vi "Create HTML.vi"(7 "FP Reference":refnum<class "Web Front Panel.lvclass">, 8 "error in (no error)":errorcluster, 10 "VI Identifier":string, 11 "Cluster In":refnum<class "Cluster.lvclass">) -> (0 "error out":errorcluster, 1 "js code for controls":string, 2 "js variables":string, 3 "Cluster Out":refnum<class "Cluster.lvclass">, 4 "script dependencies":string[](array[string]), 5 "HTML":string, 6 "js code for indicators":string)   [LabVIEW 2017, in "Front Panel Publisher.lvlib" / "Cluster.lvclass"]
uses:
  Cluster.lvclass
  C:/Backsave/Web2/FP Publisher/Front Panel Objects/Object_class/Object.lvclass
  C:/Backsave/Web2/FP Publisher/Front Panel Objects/Control_class/Control.lvclass
  Web Front Panel_class/Web Front Panel.lvclass
  Object_class/Object.lvclass
  Control_class/Control.lvclass
  <userlib>/_OpenG.lib/array/array.llb/Remove Duplicates from 1D Array (String)__ogtk.vi
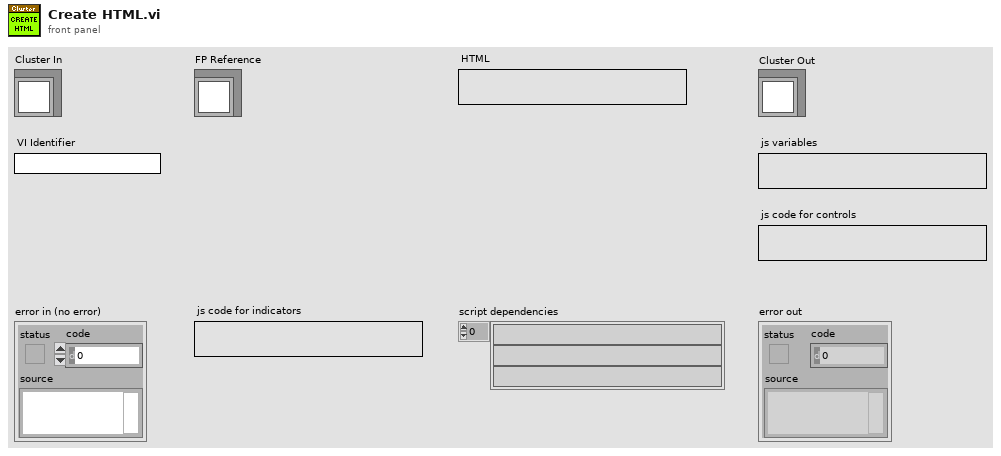
[diagram p1: front panel]
types:
  T1 = typedef "Front Panel Publisher.lvlib/Object.lvclass/Attributes.ctl" = cluster{"UID":i32, "Type":string, "Starting Location":T2, "Reference":refnum<vi>, "Cluster Component":bool, "Starting Rect Position":cluster{"Left":i16, "Top":i16}, "Owning Pane":refnum<vi>, "Master Total Rect Delta":T3}
  T2 = typedef "Front Panel Publisher.lvlib/Object.lvclass/Coordinates.ctl" = cluster{"Left":i32, "Top":i32, "Height":u32, "Width":u32}
  T3 = typedef "LVRectTypeDef.ctl" = cluster{"Left":i16, "Top":i16, "Right":i16, "Bottom":i16}
  T4 = typedef "Front Panel Publisher.lvlib/Control.lvclass/Attributes.ctl" = cluster{"Description":string, "Indicator":bool, "Default Value":variant, "Control Index":i32, "Label":refnum<class "Text.lvclass">, "Caption":refnum<class "Text.lvclass">, "Image b64":string, "No Control Index":bool, "Display Mode":T5}
  T5 = typedef "Front Panel Publisher.lvlib/Web Front Panel.lvclass/Enum - Control Display Mode.ctl" = enum16{"Value Only", "Value and Visibility", "Boolean Value Only", "Boolean Value and Visibility", "Control is Image", "Image and Visibility"}
  T6 = typedef "Front Panel Publisher.lvlib/Cluster.lvclass/Attributes.ctl" = cluster{"Cluster Decoration":refnum<class "Object.lvclass">, "Cluster Objects":refnum<class "Object.lvclass">[]}
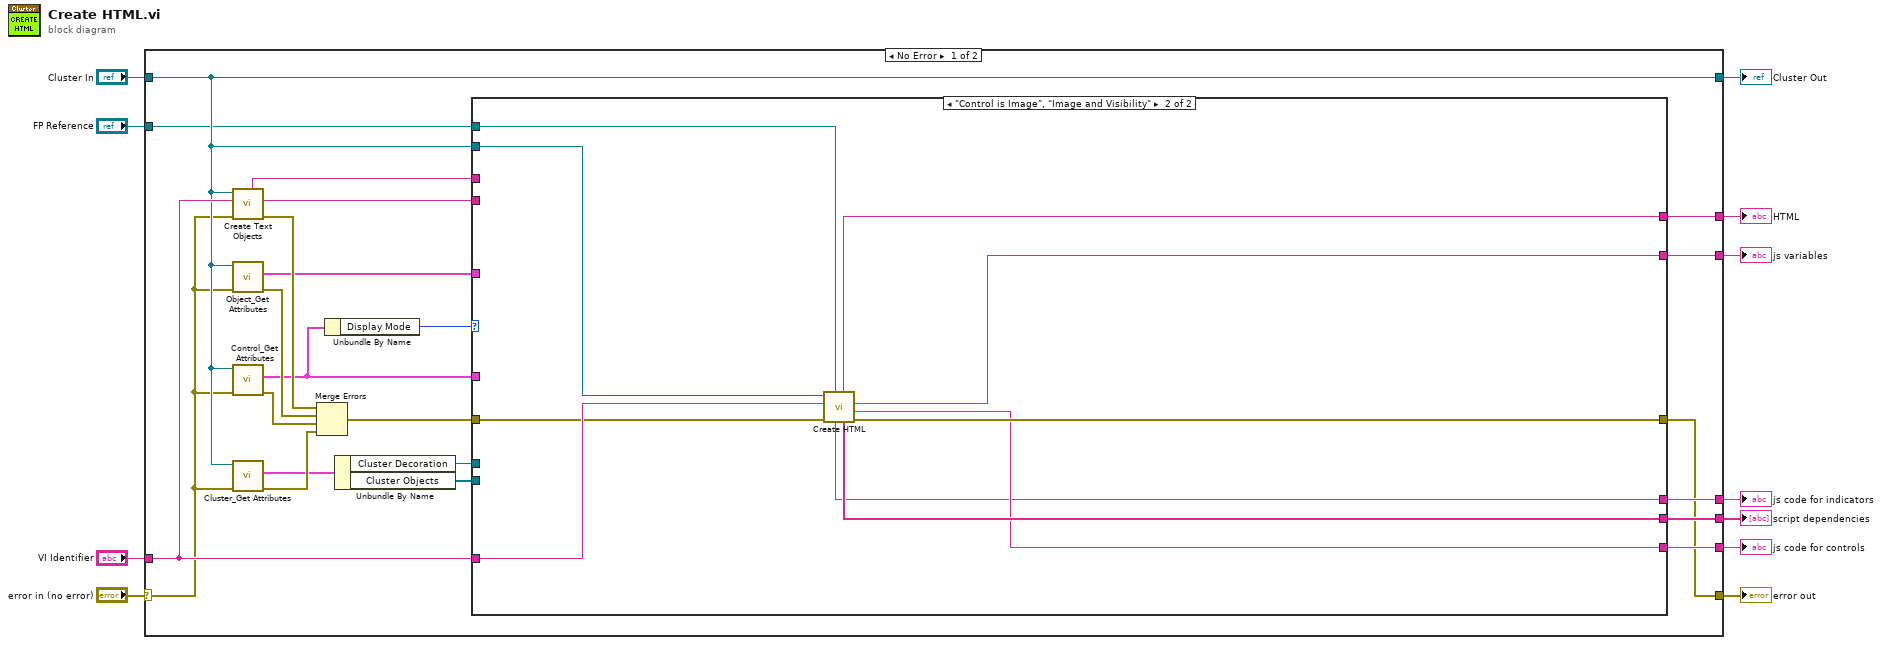
[diagram p0: block diagram]
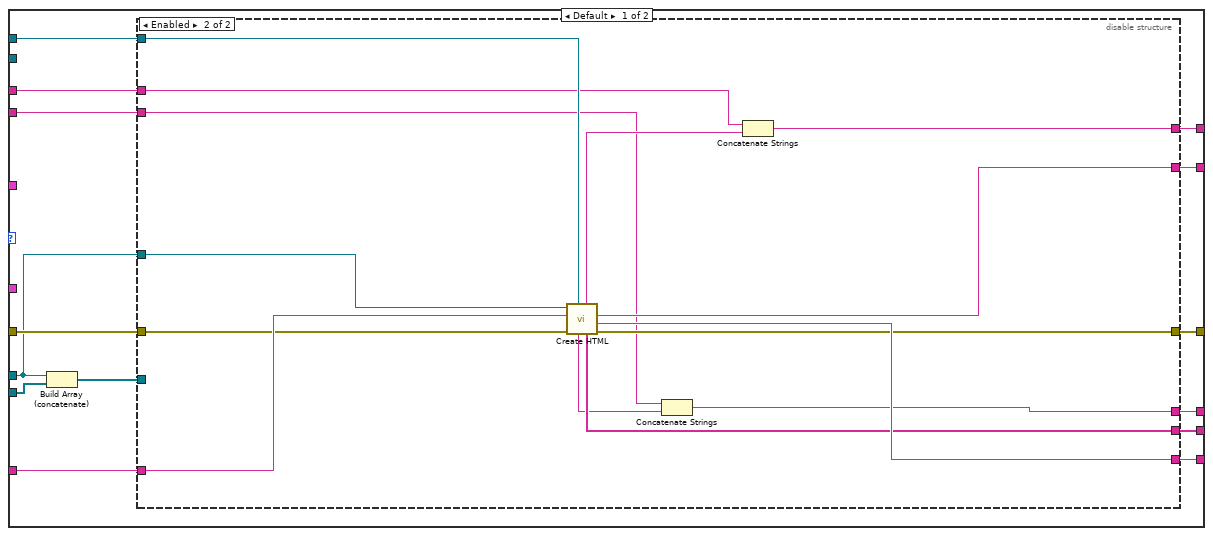
[diagram p2: hidden frame]
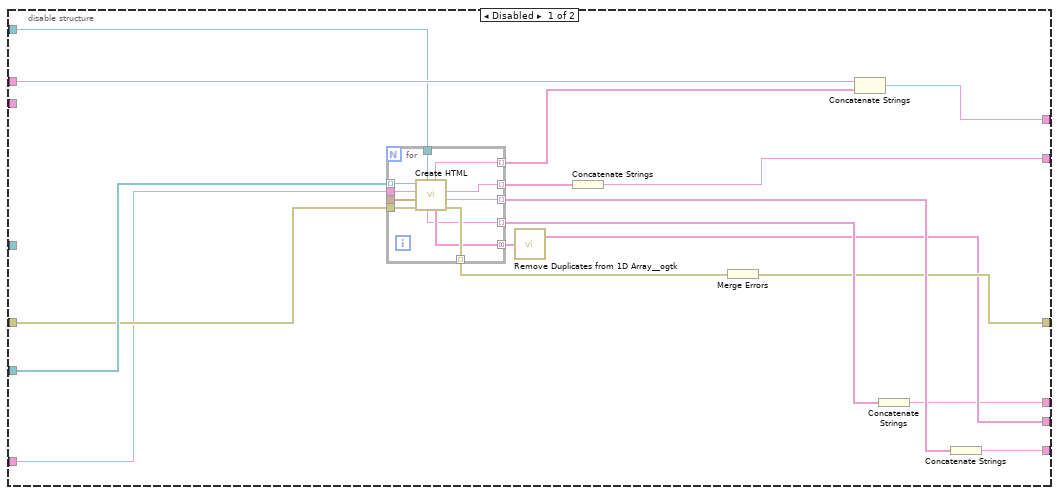
[diagram p3: hidden frame]
diagram:
  n1 = case shown="No Error" "error in (no error)" {
    selector: "error in (no error)" -> [w18 w103]
    tunnel: [w24 w103] -> w10
    tunnel: [w19 w102] -> w8
    tunnel: "Cluster In" -> [w19 w102]
    tunnel: [w31 _] -> w7
    tunnel: [w29 _] -> w6
    tunnel: [w30 _] -> w5
    tunnel: "VI Identifier" -> [w28 _]
    tunnel: [w26 _] -> w3
    tunnel: [w25 _] -> w2
    tunnel: "FP Reference" -> [w12 _]
    frame No Error {
      n2 = call-dynamic "Create Text Objects.vi"("error in (no error)"=w18, "VI Name"=w28, "Control In"=w19) -> ("error out"=w32:errorcluster, "JS Indicator"=w21:string, "HTML"=w14:string)  [unwired: 5 in, 1 out]
      n3 = call "Object_Get Attributes.vi"("error in (no error)"=w18, "Object In"=w19) -> ("error out"=w33:errorcluster, "Object Attributes"=w20:T1)  [unwired: 7 in, 1 out]
      n4 = call "Control_Get Attributes.vi"("error in (no error)"=w18, "Control In"=w19) -> ("error out"=w34:errorcluster, "Control Attributes"=w23:T4)  [unwired: 7 in, 1 out]
      n5 = call "Cluster_Get Attributes.vi"("error in (no error)"=w18, "Cluster In"=w19) -> ("error out"=w17:errorcluster, "Cluster Attributes"=w16:T6)  [unwired: 7 in, 1 out]
      n6 = Merge Errors(w32, w33, w34, w17) -> (w27:errorcluster)
      n7 = Unbundle By Name(w23) -> ("Display Mode"=w22:T5)
      n8 = Unbundle By Name(w16) -> ("Cluster Decoration"=w15:refnum<class "Object.lvclass">, "Cluster Objects"=w13:refnum<class "Object.lvclass">[])
      n9 = case shown="\"Control is Image\", \"Image and Visibility\"" w22 {
        tunnel: [w47 w96] -> w31
        tunnel: w20 -> [_ _]
        tunnel: w23 -> [_ _]
        tunnel: [w38 w94] -> w30
        tunnel: [w39 w93] -> w29
        tunnel: w14 -> [w48 _]
        tunnel: w28 -> [w37 w100]
        tunnel: w19 -> [_ w101]
        tunnel: w27 -> [w43 w99]
        tunnel: [w40 w97] -> w26
        tunnel: [w41 w95] -> w25
        tunnel: [w42 w98] -> w24
        tunnel: w21 -> [w35 _]
        tunnel: w15 -> [w36 _]
        tunnel: w13 -> [w46 _]
        tunnel: w12 -> [w44 w92]
        frame Default {
          n10 = Build Array (concatenate)(w36, w46) -> (w45:refnum<class "Object.lvclass">[])
          n11 = disable-structure shown="Enabled" {
            disable-tunnel: w48 -> [w66 w88]
            disable-tunnel: [w65 w86] -> w47
            disable-tunnel: w45 -> [w60 _]
            disable-tunnel: w44 -> [w59 w90]
            disable-tunnel: w43 -> [w57 w80]
            disable-tunnel: [w55 w81] -> w42
            disable-tunnel: [w53 w85] -> w41
            disable-tunnel: [w52 w83] -> w40
            disable-tunnel: [w51 w79] -> w39
            disable-tunnel: [w50 w84] -> w38
            disable-tunnel: w37 -> [w49 w89]
            disable-tunnel: w36 -> [_ w91]
            disable-tunnel: w35 -> [_ w78]
            frame Disabled {
              n12 = for {
                tunnel: w60 -> [w75] mode=indexing
                tunnel: [w74] -> w54 mode=indexing
                tunnel: [w73] -> w64 mode=indexing
                tunnel: [w72] -> w63 mode=indexing
                tunnel: [w71] -> w62 mode=concatenating
                tunnel: w57 -> [w77]
                tunnel: [w76] -> w56 mode=indexing
                tunnel: [w70] -> w61 mode=indexing
                tunnel: w49 -> [w69]
                tunnel: w59 -> [w68]
                tunnel: [w67] -> w58
                n13 = call-dynamic "Create HTML.vi"("FP Reference"=w68, "error in (no error)"=w77, 9:w67, "VI Identifier"=w69, "Object In"=w75) -> ("error out"=w76:errorcluster, "js code for controls"=w72:string, "js variables"=w73:string, "script dependencies"=w71:string[], "HTML"=w74:string, "js code for indicators"=w70:string)  [unwired: 1 out]
              }
              n14 = call-poly <userlib>:"Remove Duplicates from 1D Array__ogtk.vi"("Input Array"=w62) -> ("Output Array"=w52:string[])  [unwired: 1 out]
              n15 = Concatenate Strings(w64) -> (w53:string)
              n16 = Merge Errors(w56) -> (w55:errorcluster)
              n17 = Concatenate Strings(w66, w54) -> (w65:string)
              n18 = Concatenate Strings(w61) -> (w51:string)
              n19 = Concatenate Strings(w63) -> (w50:string)
            }
            frame Enabled {
              n20 = call-dynamic "Create HTML.vi"("FP Reference"=w90, "error in (no error)"=w80, "VI Identifier"=w89, "Object In"=w91) -> ("error out"=w81:errorcluster, "js code for controls"=w84:string, "js variables"=w85:string, "script dependencies"=w83:string[], "HTML"=w87:string, "js code for indicators"=w82:string)  [unwired: 1 in, 1 out]
              n21 = Concatenate Strings(w78, w82) -> (w79:string)
              n22 = Concatenate Strings(w88, w87) -> (w86:string)
            }
          }
        }
        frame "Control is Image", "Image and Visibility" {
          n23 = call-parent "Create HTML.vi"("FP Reference"=w92, "error in (no error)"=w99, "VI Identifier"=w100, "Control In"=w101) -> ("error out"=w98:errorcluster, "js code for controls"=w94:string, "js variables"=w95:string, "script dependencies"=w97:string[], "HTML"=w96:string, "js code for indicators"=w93:string)  [unwired: 1 in, 1 out]
        }
      }
    }
    frame Error {
    }
  }
  "error out" <- w10
  "Cluster Out" <- w8
  "HTML" <- w7
  "js variables" <- w2
  "js code for controls" <- w5
  "script dependencies" <- w3
  "js code for indicators" <- w6
